vi "2898 Ball Management.vi"(5 "Bottom Front Sensor":bool, 6 "De-Jam":bool, 7 "Shoot?":bool, 8 "# of Balls":i32, 9 "Top Ball Sensor":bool, 10 "Bottom Back Sensor":bool, 11 "Enum":enum16{"Init", "Run", "End"}(ring)) -> ()   [LabVIEW 2011]
panel:
  in  "y":dbl=40.0
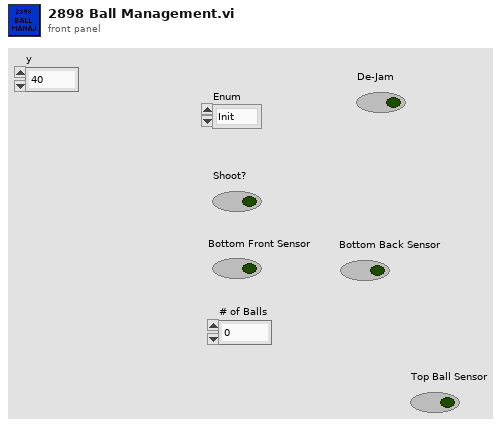
[diagram p1: front panel]
types:
  T1 = enum16{"Init", "Stop", "Collect", "Slow Collect", "Reject", "End"}
  T2 = enum16{"Init", "Stop", "Convey", "Soft Convey", "DeJam", "End"}
  T3 = enum16{"Init", "Stop", "Shoot", "Reverse", "End"}
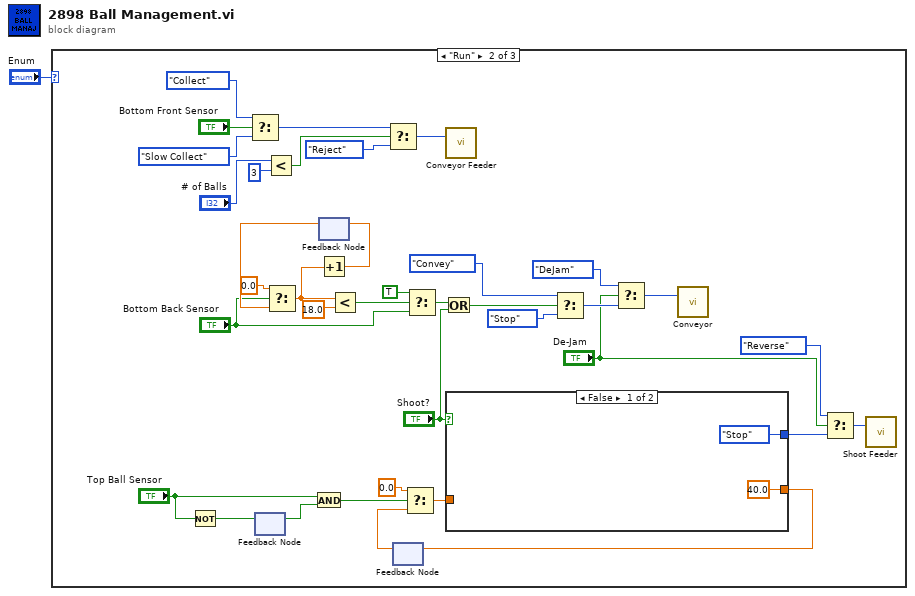
[diagram p0: block diagram]
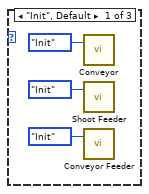
[diagram p2: hidden frame]
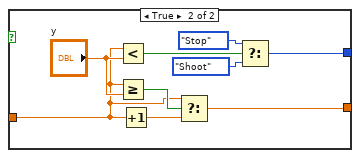
[diagram p3: hidden frame]
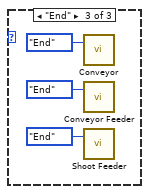
[diagram p4: hidden frame]
diagram:
  n1 = case shown="\"Run\"" "Enum" {
    frame "Init", Default {
      n2 = call "Conveyor.vi"("Enum"=T2."Init") -> ()  [unwired: 2 in]
      n3 = call "Shoot Feeder.vi"("Enum"=T3."Init") -> ()  [unwired: 2 in]
      n4 = call "Conveyor Feeder.vi"("Enum"=T1."Init") -> ()  [unwired: 2 in]
    }
    frame "Run" {
      n5 = Not(x="Top Ball Sensor") -> (.not. x?=w32:bool)
      n6 = Select(t=T1."Collect" ("Enum"), s="Bottom Front Sensor", f=T1."Slow Collect" ("Enum")) -> (s? t:f=w6:T1)
      n7 = feedback #1() -> (w26:bool)  [unwired: 1 in]
      n8 = feedback-in #1(w32) -> ()
      n9 = Less?(x="# of Balls", y=3) -> (x < y?=w20:bool)
      n10 = And(x="Top Ball Sensor", y=w26) -> (x .and. y?=w31:bool)
      n11 = feedback #2() -> (w14:dbl)  [unwired: 1 in]
      n12 = Select(t=0.0, s="Bottom Back Sensor", f=w14) -> (s? t:f=w11:dbl)
      n13 = Increment(x=w11) -> (x+1=w10:dbl)
      n14 = feedback-in #2(w10) -> ()
      n15 = Less?(x=w11, y=18.0) -> (x < y?=w12:bool)
      n16 = Select(t=w6, s=w20, f=T1."Reject") -> (s? t:f=w22:T1)
      n17 = feedback #3() -> (w29:dbl)  [unwired: 1 in]
      n18 = Select(t=0.0, s=w31, f=w29) -> (s? t:f=w28:dbl)
      n19 = Select(t=TRUE, s=w12, f="Bottom Back Sensor") -> (s? t:f=w16:bool)
      n20 = Or(x=w16, y="Shoot?") -> (x .or. y?=w19:bool)
      n21 = call "Conveyor Feeder.vi"("Enum"=w22) -> ()  [unwired: 2 in]
      n22 = case shown="False" "Shoot?" {
        tunnel: w28 -> [_ w46]
        tunnel: [40.0 w44] -> w27
        tunnel: [T3."Stop" ("Enum") w50] -> w25
        frame False {
        }
        frame True {
          n23 = Less?(x=w46, y="y") -> (x < y?=w52:bool)
          n24 = Greater Or Equal?(x=w46, y="y") -> (x >= y?=w47:bool)
          n25 = Increment(x=w46) -> (x+1=w45:dbl)
          n26 = Select(t=w46, s=w47, f=w45) -> (s? t:f=w44:dbl)
          n27 = Select(t=T3."Stop" ("Enum"), s=w52, f=T3."Shoot") -> (s? t:f=w50:T3)
        }
      }
      n28 = feedback-in #3(w27) -> ()
      n29 = Select(t=T2."Convey" ("Enum"), s=w19, f=T2."Stop" ("Enum")) -> (s? t:f=w38:T2)
      n30 = Select(t=T2."DeJam" ("Enum"), s="De-Jam", f=w38) -> (s? t:f=w36:T2)
      n31 = call "Conveyor.vi"("Enum"=w36) -> ()  [unwired: 2 in]
      n32 = Select(t=T3."Reverse", s="De-Jam", f=w25) -> (s? t:f=w23:T3)
      n33 = call "Shoot Feeder.vi"("Enum"=w23) -> ()  [unwired: 2 in]
    }
    frame "End" {
      n34 = call "Conveyor.vi"("Enum"=T2."End") -> ()  [unwired: 2 in]
      n35 = call "Conveyor Feeder.vi"("Enum"=T1."End") -> ()  [unwired: 2 in]
      n36 = call "Shoot Feeder.vi"("Enum"=T3."End") -> ()  [unwired: 2 in]
    }
  }
